vi "Versuchsaufbau bearbeiten.vi"(6 "error in (no error)":errorcluster, 8 "Setup in":refnum<class "Setup.lvclass">, 9 "Data":T1={"Report.lvclass"=refnum, "Norm"="", "last State"=enum."Initialize", "Norm ID"=0, "EMTestCWS500N.lvclass"=refnum, "CEG4500.lvclass"=refnum, "Tektronix RSA5106A.lvclass"=refnum, "erfolgreich"=FALSE, "Device Enum"=enum."emTestCWS500N", "Test Enum"=enum."ESD", "debug"=FALSE, "tab"=enum."Hauptmenü", "ESD Pistol.lvclass"=refnum, "SubPnl Refnum"=refnum, "TabCtl Refnum"=refnum, "ButtonsEinblenden?"=FALSE, "VKey"=enum."ASCII", "last Test"=refnum}) -> (0 "error out 2":errorcluster caption="error out", 2 "Setup Ausgang":refnum<class "Setup.lvclass">, 3 "Abbrechen out":bool)   [LabVIEW 2013, in "DataCreation.lvlib"]
doc: "Hier wird der Versuchsaufbau dokumentiert. Es gibt die Möglichkeit Bilder und die genutzten Geräte zu hinterlegen. Mit diesem VI kann auch ein bestehender Versuchsaufbau bearbeitet werden, in diesem Fall wird ein Setup-Objekt als Eingabe benötigt.\nNach korrekter Ausführung wird ein Setup-Objekt zurückgegeben das einem Norm-Objekt zugeordnet werden kann."
uses:
  lib/DataCreation.lvlib
  Main/controls/Data.ctl
  classes/Datastructure/Report/Report.lvclass
  classes/Devices/emTestCWS500N/EMTestCWS500N.lvclass
  classes/Devices/CEG4500/CEG4500.lvclass
  classes/Devices/Tektronix RSA5106A/Tektronix RSA5106A.lvclass
  ESD Pistol.lvclass
  classes/Datastructure/Test/Test.lvclass
  Main/controls/State.ctl
  classes/Devices/DeviceInterface/Devices.ctl
  classes/Tests/TestInterface/Tests.ctl
  Tabs.ctl
  <vilib>/event_ctls.llb/eventvkey.ctl
  classes/Datastructure/Setup/Setup.lvclass
  SetupData2.ctl
  classes/Datastructure/Device/Device.lvclass
  classes/Datastructure/Image/img.lvclass
  <vilib>/regexp/Match Regular Expression.xnode
  lib/TreeRepresentation.lvlib
panel:
  in  "dev id":i32
  in  "pic id":i32
  in  "Tab Control":enum32{"Versuchsaufbau", "Daten"}(tab)
  in  "Abbrechen":bool
  in  "Tree pics & devs":string(tree)
  out "Titel":string caption="Test"
  in  "OK Button":bool
  in  "Add picture":bool
  in  "Kommentar":string
  in  "Add Device":bool
  in  "Tree Report":string(tree)
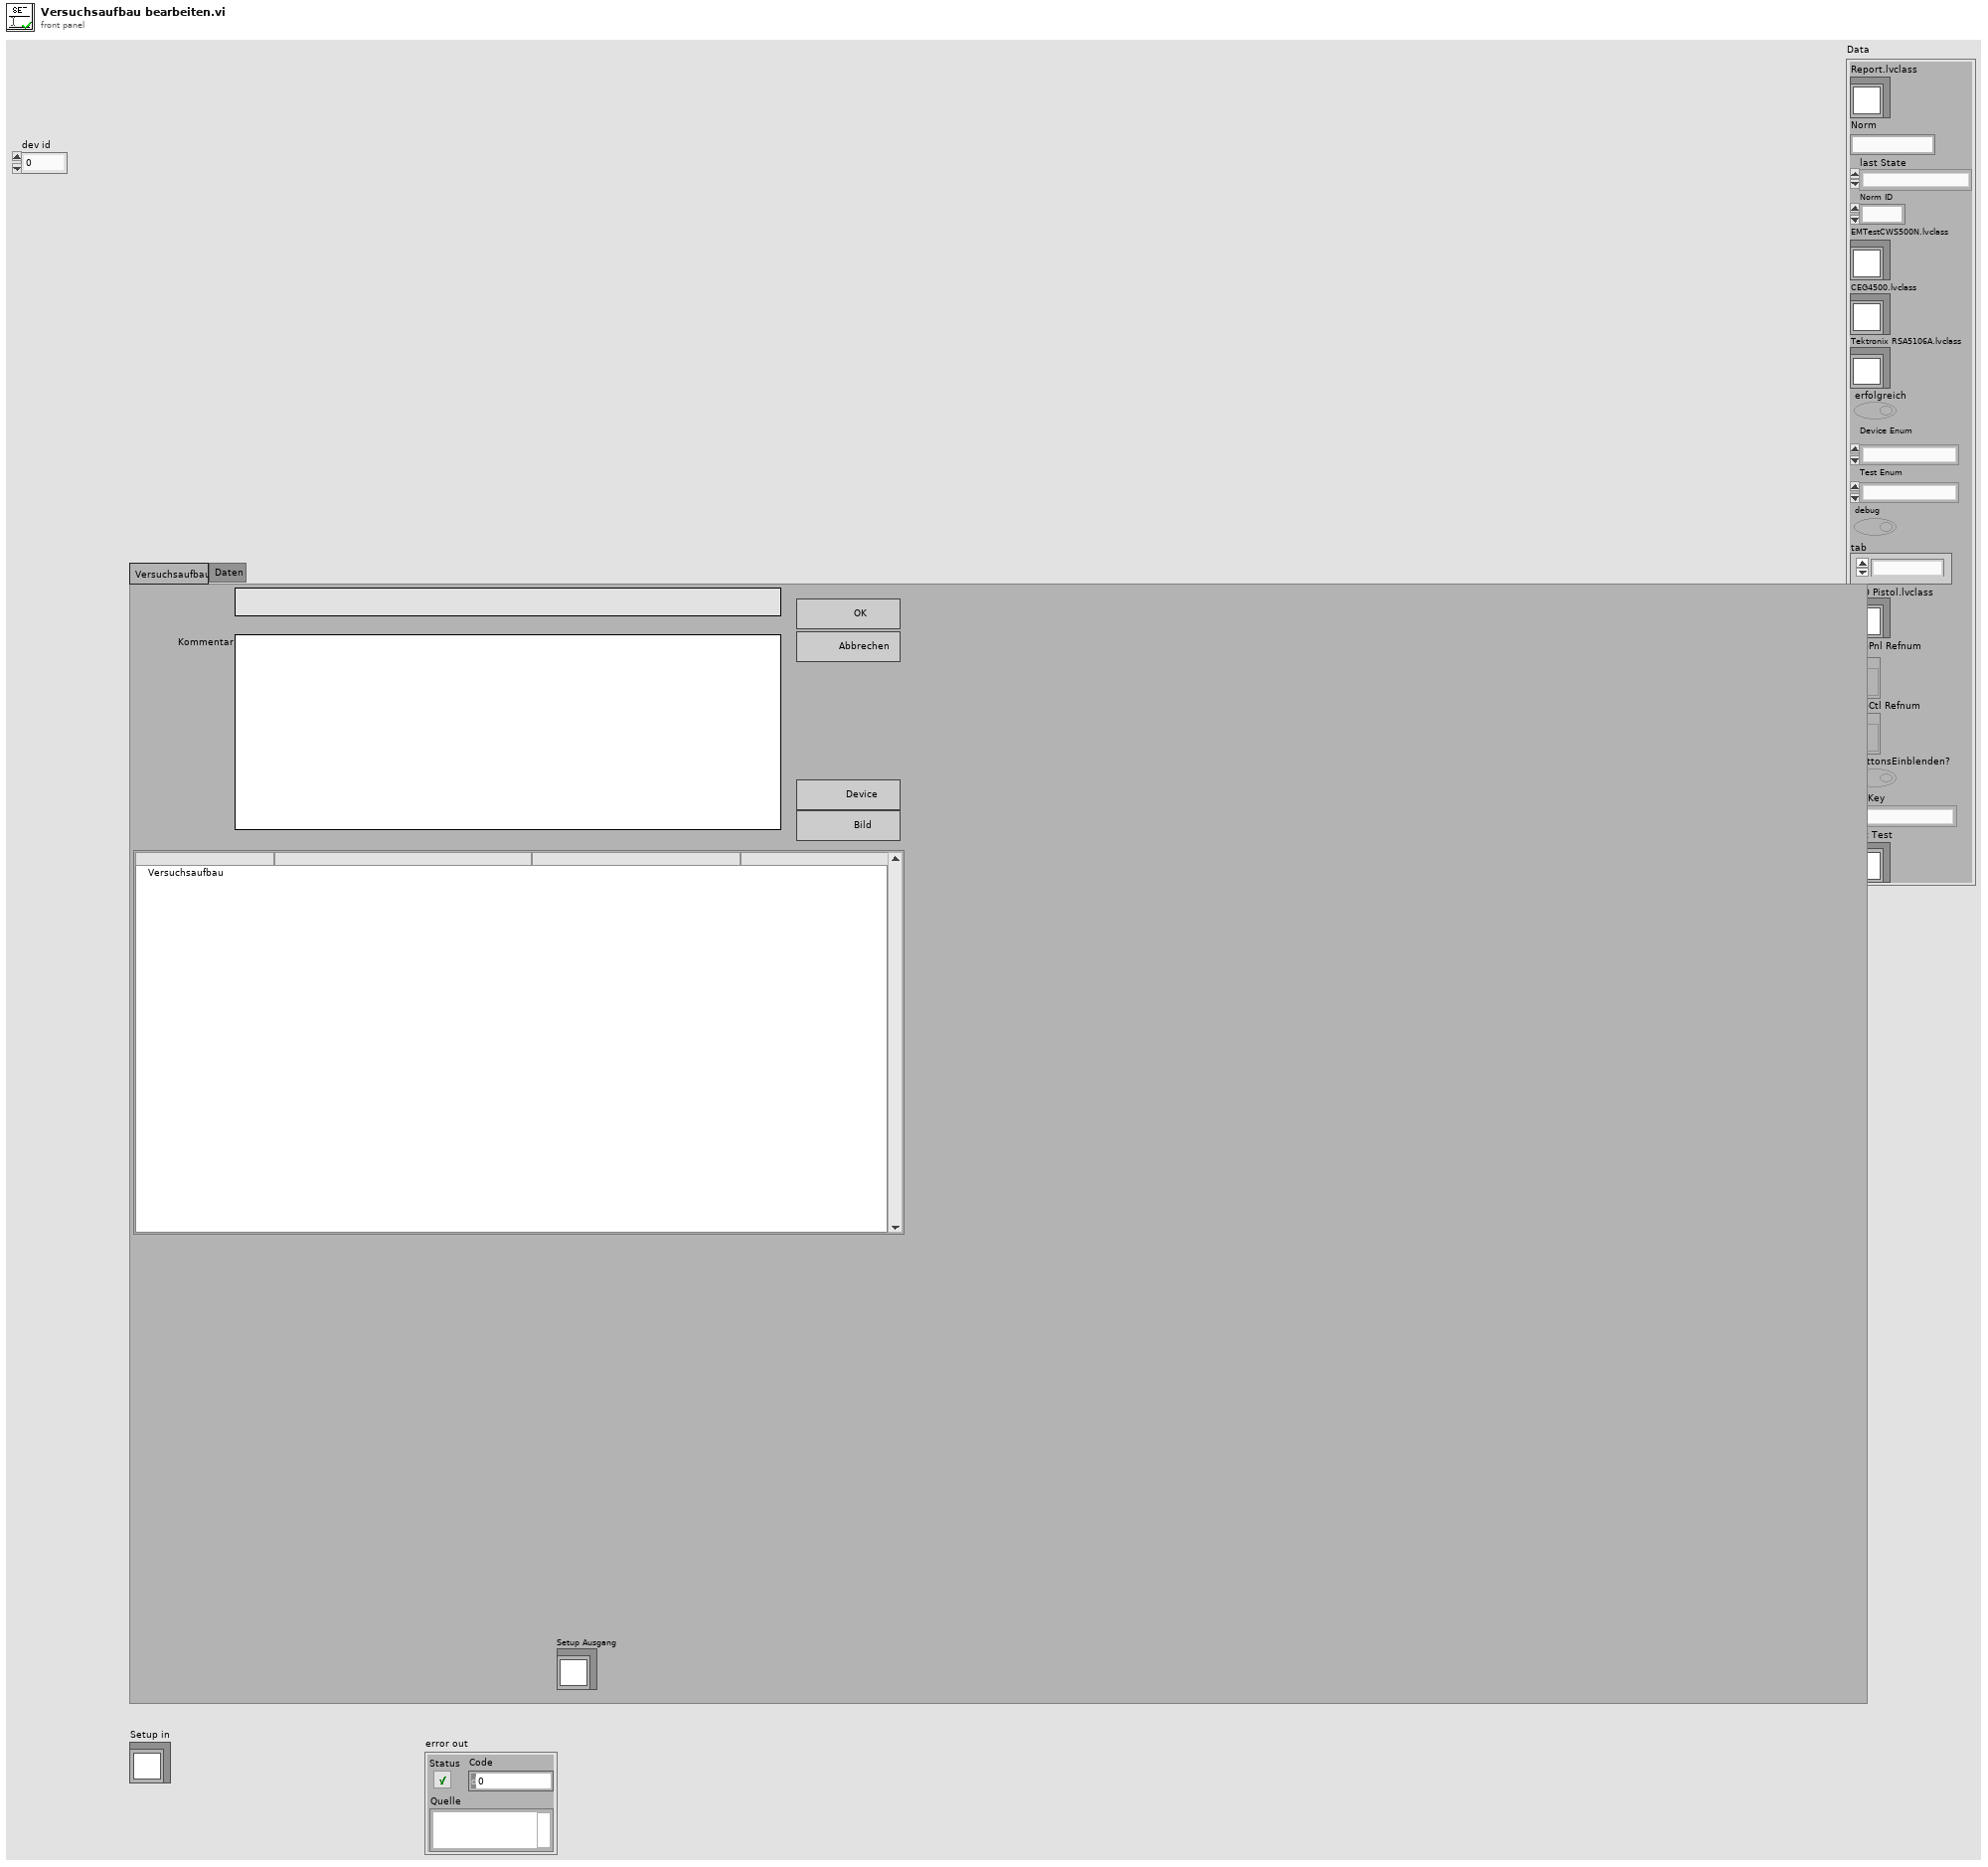
[diagram p1: front panel]
types:
  T1 = typedef "Data.ctl" = cluster{"Report.lvclass":refnum<class "Report.lvclass">, "Norm":string, "last State":T2, "Norm ID":i32, "EMTestCWS500N.lvclass":refnum<class "EMTestCWS500N.lvclass">, "CEG4500.lvclass":refnum<class "CEG4500.lvclass">, "Tektronix RSA5106A.lvclass":refnum<class "Tektronix RSA5106A.lvclass">, "erfolgreich":bool, "Device Enum":T3, "Test Enum":T4, "debug":bool, "tab":T5, "ESD Pistol.lvclass":refnum<class "ESD Pistol.lvclass">, "SubPnl Refnum":refnum<vi>, "TabCtl Refnum":refnum<vi>, "ButtonsEinblenden?":bool, "VKey":T6, "last Test":refnum<class "Test.lvclass">}
  T2 = typedef "State.ctl" = enum16{"create Pdf", "edit Report", "load Report", "save Report", "do Test", "CDN Kalibrierung", "enter Report Parameters", "new Test", "Protokoll", "read Tree", "update Tree", "Fehler", "Initialize", "Wait for Event", "Exit"}
  T3 = typedef "Devices.ctl" = enum16{"unbekannt", "ESD Pistol", "Tektronix RSA5106A", "emTestCWS500N", "CEG-4500"}
  T4 = typedef "Tests.ctl" = enum16{"unbekannt", "Störaussendung", "Burst", "ESD", "Surge", "Spannungseinbruch", "HF-Felder"}
  T5 = typedef "Tabs.ctl" = enum32{"Hauptmenü", "Prüfbericht", "Einstellungen"}
  T6 = typedef "eventvkey.ctl" = enum16{"ASCII", "Enter", "Return", "Shift", "Ctrl", "Alt", "Cmd", "Opt", "Caps", "NumLock", "Clear", "Break", "Up", "Down", "Left", "Right", "Insert", "Delete", "Home", "End", "PageUp", "PageDown", "Escape", "Help", "Pause", "ScrollLock", "F1", "F2", "F3", "F4", "F5", "F6", "F7", "F8", "F9", "F10", "F11", "F12", "F13", "F14", "F15", "F16", "F17", "F18", "F19", "F20", "F21", "F22", "F23", "F24", "Play", "VolumeUp", "VolumeDown", "Mute", "Two Byte Char"}
  T7 = typedef "DataCreation.lvlib/SetupData2.ctl" = cluster{"Device":refnum<class "Device.lvclass">, "img":refnum<class "img.lvclass">, "tag":string, "editDev":bool}
  T8 = enum16{"add pic", "add dev", "ok", "abbrechen", "wait for event"}
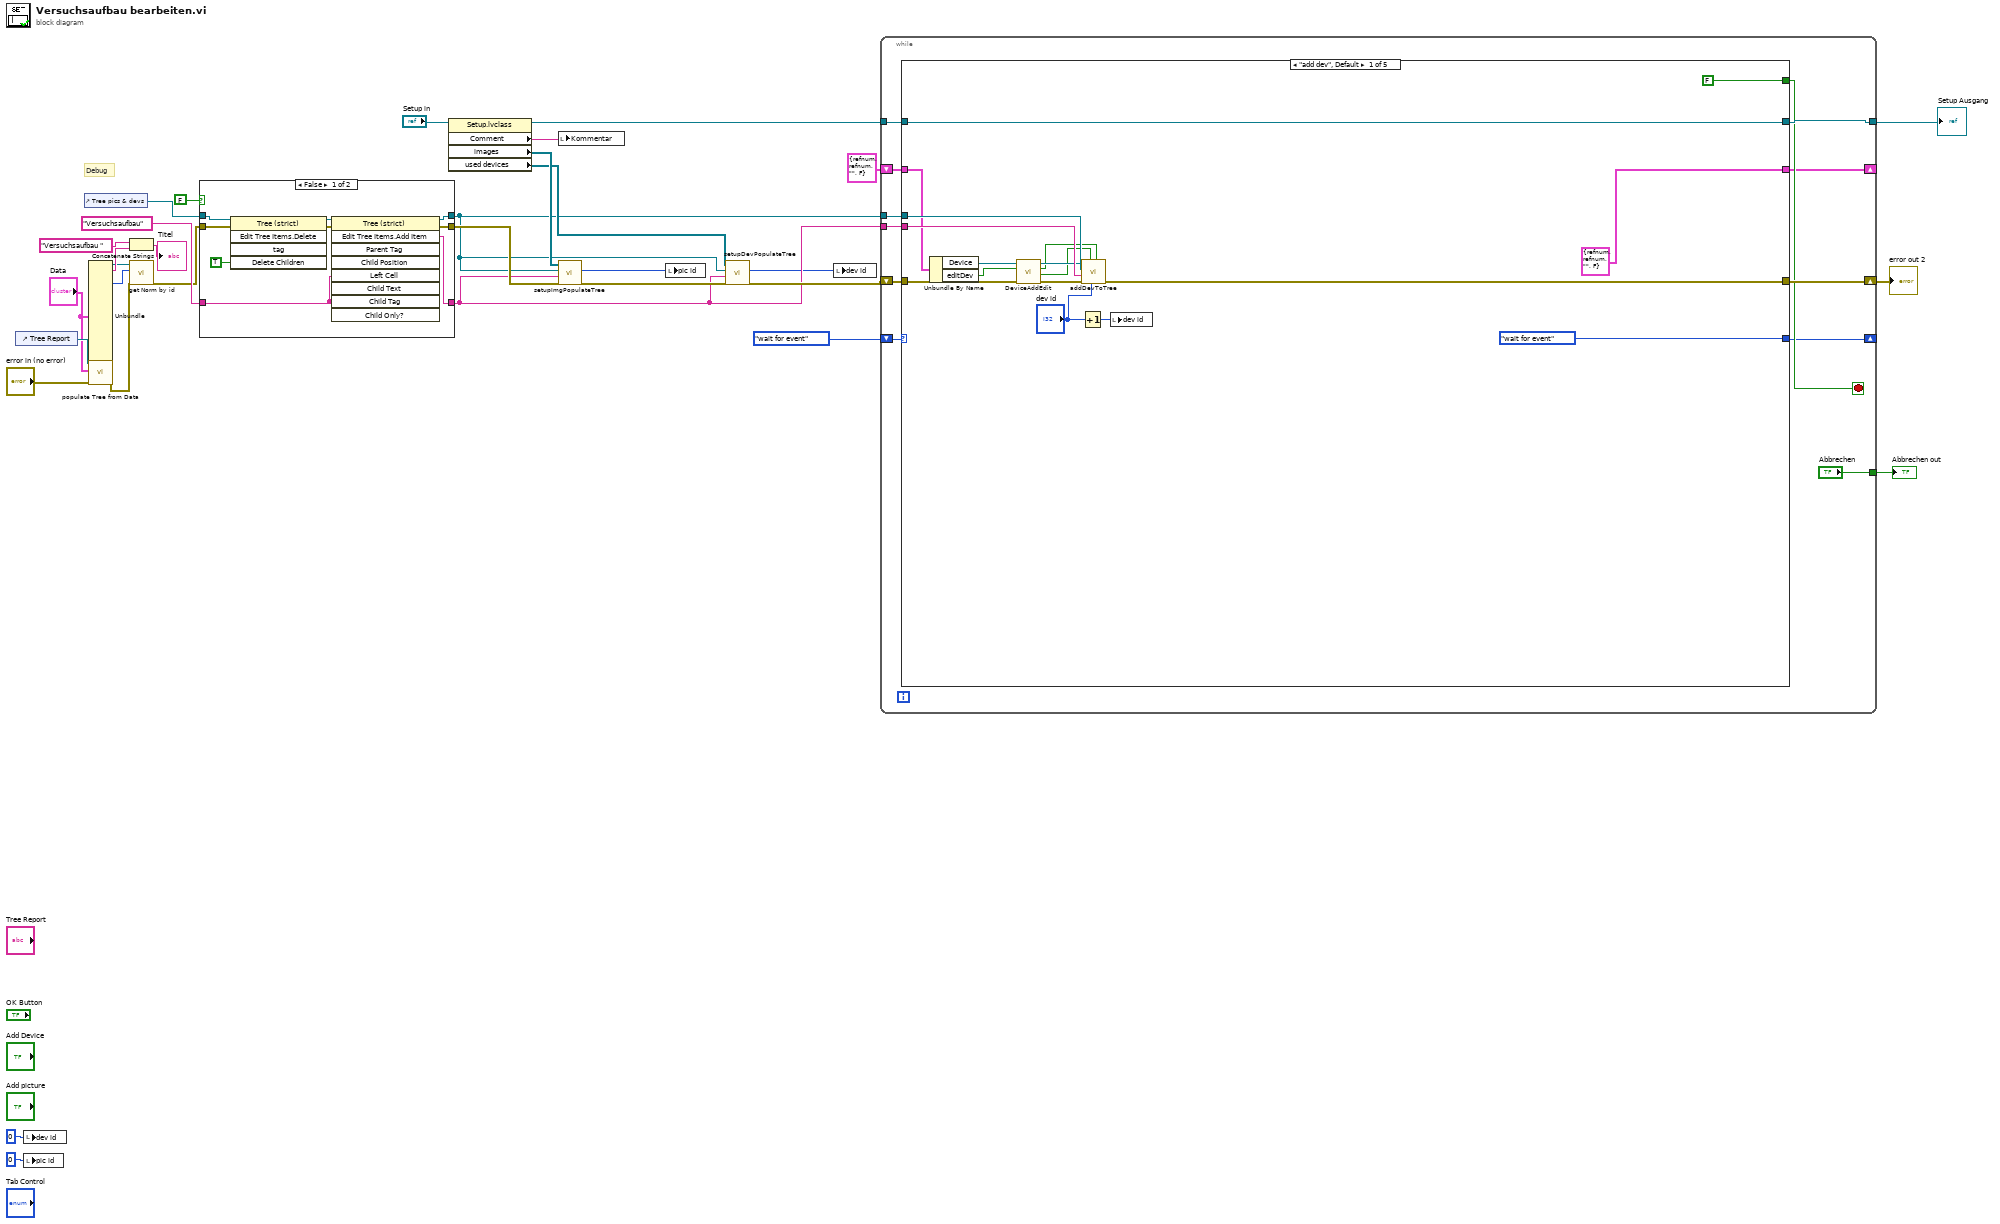
[diagram p0: block diagram]
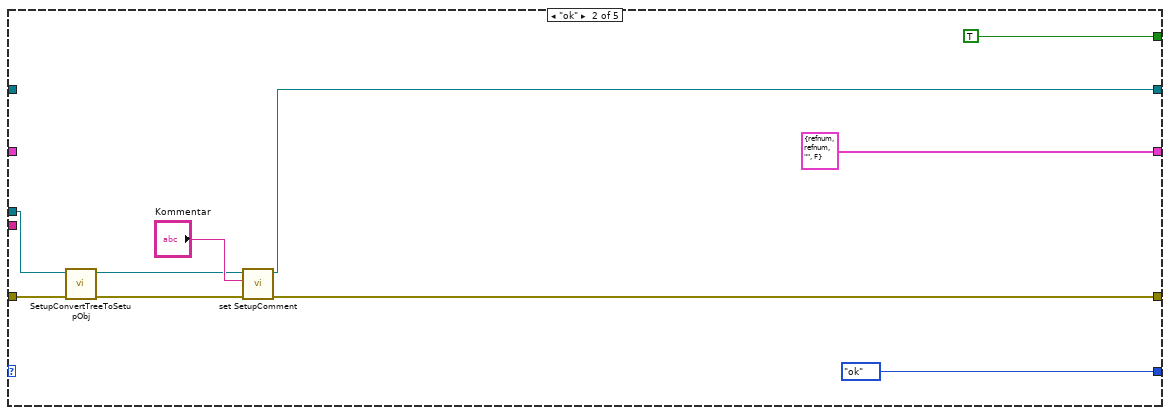
[diagram p3: hidden frame]
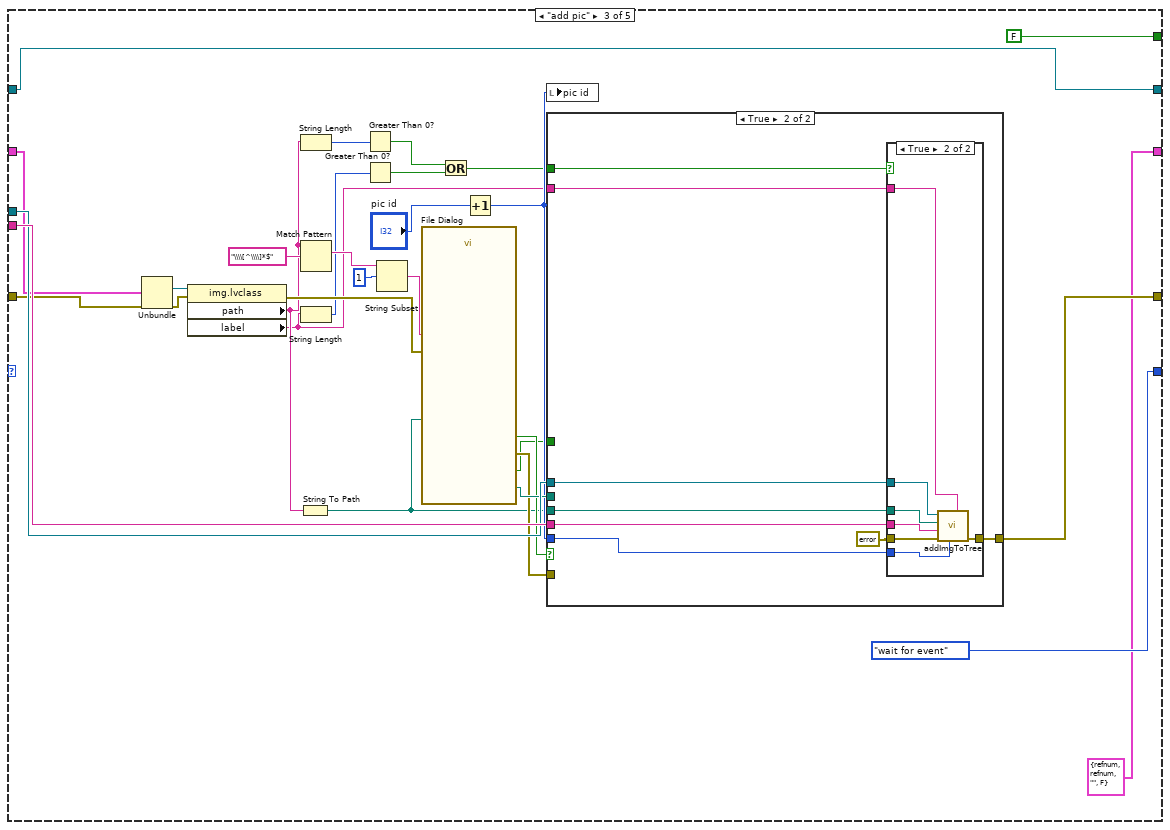
[diagram p4: hidden frame]
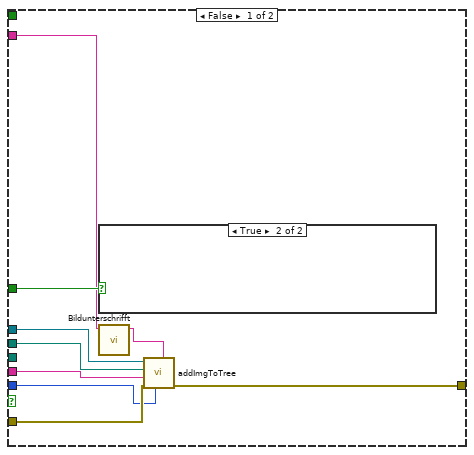
[diagram p5: hidden frame]
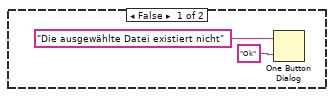
[diagram p6: hidden frame]
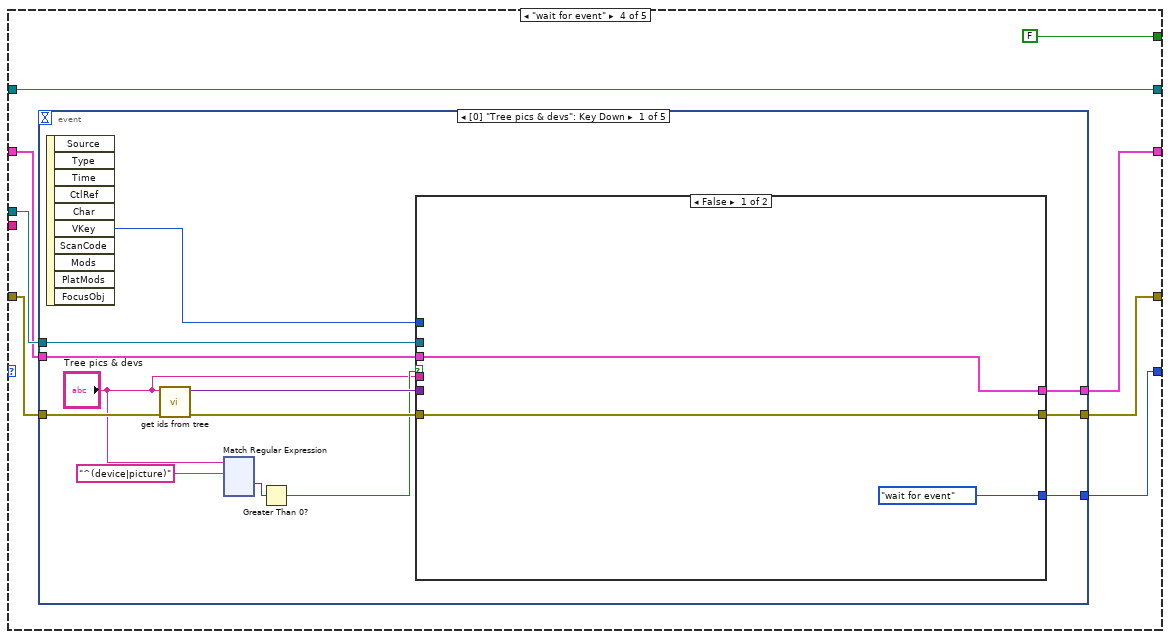
[diagram p8: hidden frame]
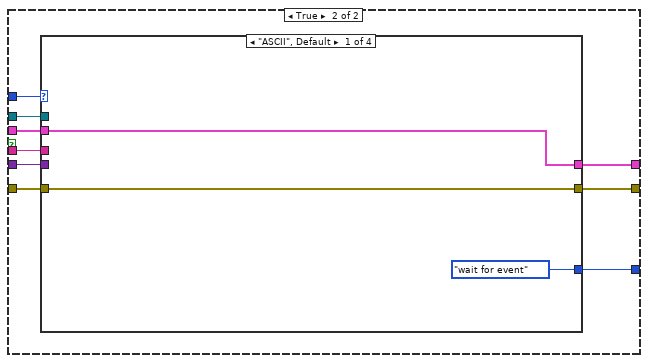
[diagram p9: hidden frame]
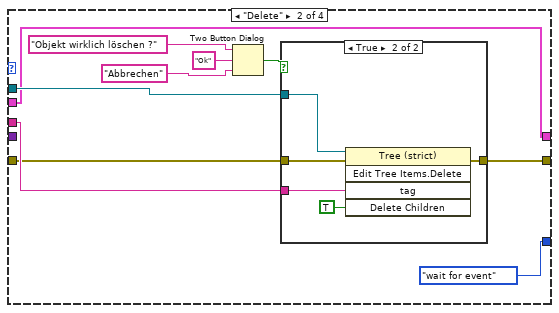
[diagram p10: hidden frame]
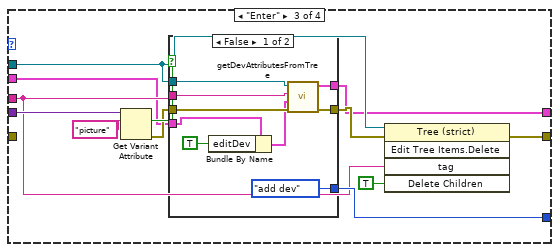
[diagram p12: hidden frame]
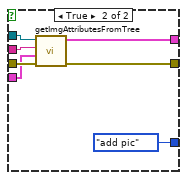
[diagram p13: hidden frame]
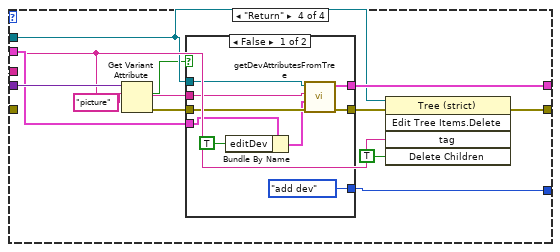
[diagram p14: hidden frame]
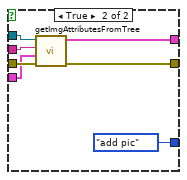
[diagram p15: hidden frame]
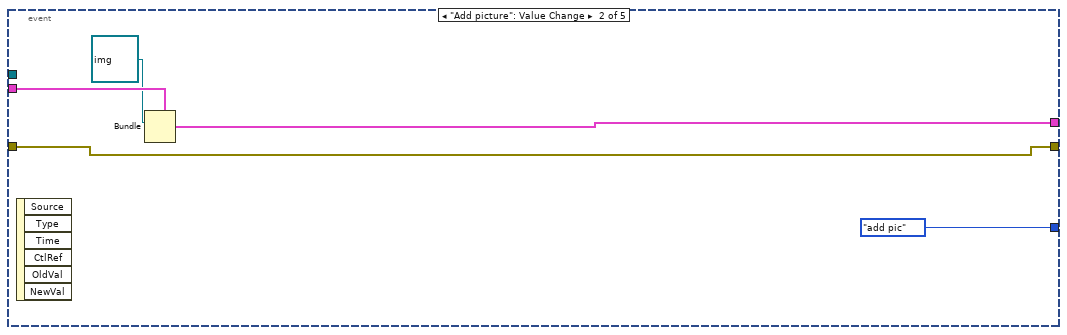
[diagram p16: hidden frame]
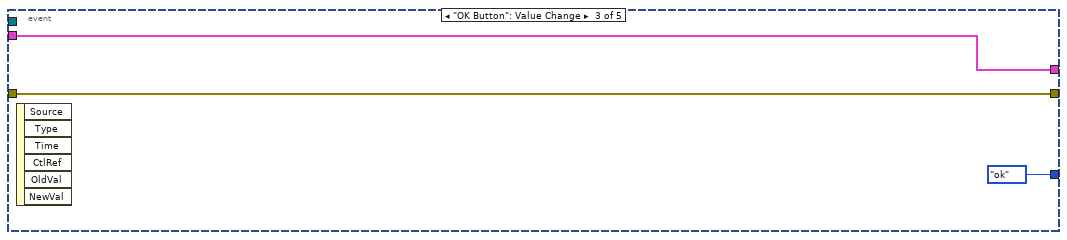
[diagram p17: hidden frame]
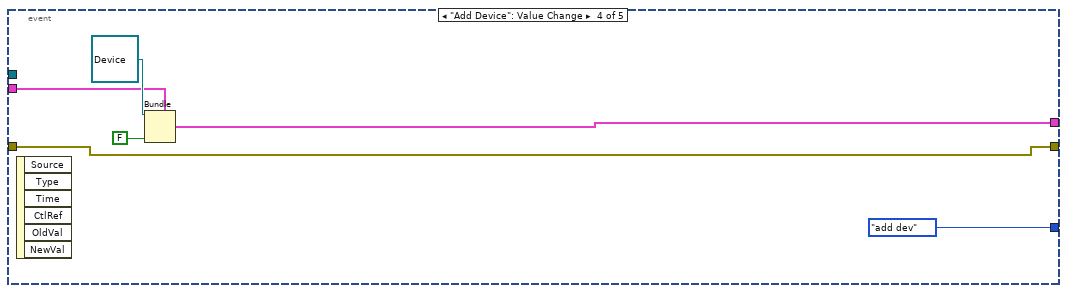
[diagram p18: hidden frame]
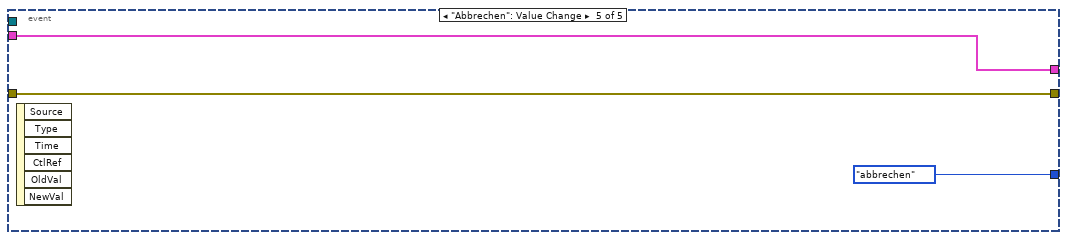
[diagram p19: hidden frame]
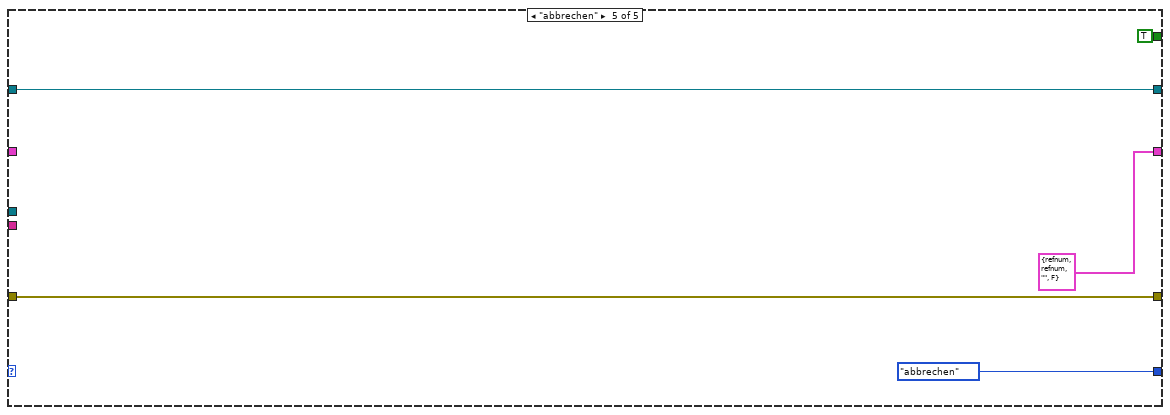
[diagram p20: hidden frame]
diagram:
  # "Debug"
  n1 = control-ref of="Tree Report"() -> (w32:refnum<vi>)
  n2 = local write "dev id"(0 ("number of devices")) -> ()
  n3 = local write "pic id"(0 ("number of devices")) -> ()
  n4 = control-ref of="Tree pics & devs"() -> (w21:refnum<vi>)
  n5 = Unbundle("Data") -> ("Report.lvclass"=w27:refnum<class "Report.lvclass">, "Norm"=w28:string, "Norm ID"=w24:i32)  [unwired: 15 out]
  n6 = call "populate Tree from Data.vi"("error in (no error)"="error in (no error)", "Data"="Data", "reference"=w32) -> ("error out"=w26:errorcluster)  [unwired: 6 in]
  n7 = Concatenate Strings("Versuchsaufbau ", w28) -> (→"Titel":string)
  n8 = call-dynamic "get Norm by id.vi"("error in (no error)"=w26, "id"=w24, "Report (Eingang)"=w27) -> ("error out"=w22:errorcluster)  [unwired: 4 in, 4 out]
  n9 = case shown="False" FALSE {
    tunnel: "Versuchsaufbau" ("Elternobjekt-Tag") -> [w41 w42]
    tunnel: [w40 w42] -> w10
    tunnel: [w39 w44] -> w15
    tunnel: w22 -> [w38 w44]
    tunnel: w21 -> [w37 w43]
    tunnel: [w36 w43] -> w8
    frame False {
      n10 = invoke on="Invoke Node" class="Tree (strict)" method="Edit Tree Items.Delete"(reference=w37, error in=w38, "Delete Children"=TRUE ("Unterobjekte löschen?")) -> (reference out=w35:refnum<vi>, error out=w34:errorcluster)  [unwired: 2 in, 3 out]
      n11 = invoke class="Tree (strict)" method="Edit Tree Items.Add Item"(reference=w35, error in=w34, "Left Cell"=w41, "Child Tag"=w41) -> (reference out=w36:refnum<vi>, error out=w39:errorcluster, "Edit Tree Items:Add Item"=w40:string)  [unwired: 5 in, 6 out]
    }
    frame True {
    }
  }
  n12 = property class="Setup.lvclass"(reference="Setup in") -> (reference out=w5:refnum<class "Setup.lvclass">, "Comment"=w16:string, "images"=w13:refnum<class "img.lvclass">[], "used devices"=w9:refnum<class "Device.lvclass">[])  [unwired: 1 in, 1 out]
  n13 = local write "Kommentar"(w16) -> ()
  n14 = call "setupImgPopulateTree.vi"("error in (no error)"=w15, "Elternobjekt-Tag"=w10, "Tree in"=w8, "images"=w13) -> ("error out"=w12:errorcluster, "#pics"=w14:i32)  [unwired: 6 in]
  n15 = local write "pic id"(w14) -> ()
  n16 = call "setupDevPopulateTree.vi"("error in (no error)"=w12, "Elternobjekt-Tag"=w10, "TreeControl in"=w8, "used devices"=w9) -> ("error out"=w11:errorcluster, "#dev"=w7:i32)  [unwired: 6 in]
  n17 = local write "dev id"(w7) -> ()
  n18 = while {
    tunnel: w10 -> [w53]
    tunnel: w8 -> [w55]
    tunnel: [w52] -> w3
    shift-right: [w51] -> w4
    shift-left: w11 -> [w56]
    shift-right: [w49] -> _
    shift-left: T8."wait for event" -> [w54]
    tunnel: w5 -> [w48]
    shift-right: [w46] -> _
    shift-left: T7 {"Device"=refnum, "img"=refnum, "tag"="", "editDev"=FALSE} -> [w47]
    tunnel: ["Abbrechen"] -> w1
    stop <- w50 stop-if-true
    n19 = case shown="\"add dev\", Default" w54 {
      tunnel: [w71 w75 w112 w141 w381] -> w51
      tunnel: w56 -> [w64 w82 w102 w142 w381]
      tunnel: w53 -> [w73 _ w111 _ _]
      tunnel: w55 -> [w72 w83 w110 w147 _]
      tunnel: [w68 w76 w105 w144 w380] -> w52
      tunnel: [FALSE TRUE FALSE FALSE TRUE] -> w50
      tunnel: [T8."wait for event" T8."ok" T8."wait for event" w145 T8."abbrechen"] -> w49
      tunnel: w48 -> [w68 _ w105 w144 w380]
      tunnel: w47 -> [w67 _ w104 w143 _]
      tunnel: [T7 {"Device"=refnum, "img"=refnum, "tag"="", "editDev"=FALSE} T7 {"Device"=refnum, "img"=refnum, "tag"="", "editDev"=FALSE} T7 {"Device"=refnum, "img"=refnum, "tag"="", "editDev"=FALSE} w140 T7 {"Device"=refnum, "img"=refnum, "tag"="", "editDev"=FALSE}] -> w46
      frame "add dev", Default {
        n20 = Unbundle By Name(w67) -> ("Device"=w66:refnum<class "Device.lvclass">, "editDev"=w57:bool)
        n21 = call "DeviceAddEdit.vi"("error in"=w64, "editDev"=w57, "Dev in"=w66) -> ("error out"=w63:errorcluster, "Dev löschen"=w62:bool, "Abbruch?"=w58:bool, "Dev out"=w65:refnum<class "Device.lvclass">)  [unwired: 5 in]
        n22 = Increment(x="dev id") -> (x+1=w59:i32)
        n23 = call "addDevToTree.vi"("abbrechen"=w58, "dev id"="dev id", "Dev löschen"=w62, "error in (no error)"=w63, "Elternobjekt-Tag"=w73, "Tree pics & devs"=w72, "Device in"=w65) -> ("error out"=w71:errorcluster)  [unwired: 4 in]
        n24 = local write "dev id"(w59) -> ()
      }
      frame "ok" {
        n25 = call "SetupConvertTreeToSetupObj.vi"("error in (no error)"=w82, "TreeControl in"=w83) -> ("error out"=w79:errorcluster, "Setup out"=w77:refnum<class "Setup.lvclass">)  [unwired: 8 in]
        n26 = call-dynamic "set SetupComment.vi"("error in (no error)"=w79, "Comment"="Kommentar", "Setup (Eingang)"=w77) -> ("error out"=w75:errorcluster, "Setup (Ausgang)"=w76:refnum<class "Setup.lvclass">)  [unwired: 7 in]
      }
      frame "add pic" {
        n27 = Unbundle(w104) -> ("img"=w103:refnum<class "img.lvclass">)  [unwired: 3 out]
        n28 = property class="img.lvclass"(reference=w103, error in=w102) -> (error out=w101:errorcluster, "path"=w93:string, "label"=w92:string)  [unwired: 1 out]
        n29 = String To Path(string=w93) -> (path=w86:path)
        n30 = String Length(string=w93) -> (length=w91:i32)
        n31 = Match Pattern(string=w93, regular expression="\\\\[^\\\\]*$") -> (match substring=w96:string)  [unwired: 1 in, 3 out]
        n32 = String Length(string=w92) -> (length=w90:i32)
        n33 = Greater Than 0?(x=w91) -> (x > 0?=w89:bool)
        n34 = Greater Than 0?(x=w90) -> (x > 0?=w88:bool)
        n35 = String Subset(string=w96, offset (0)=1) -> (substring=w94:string)  [unwired: 1 in]
        n36 = call "File Dialog"("start path"=w86, "default name"=w94, "error in"=w101) -> ("selected path"=w109:path, "exists"=w84:bool, "cancelled"=w87:bool, "error out"=w108:errorcluster)  [unwired: 9 in]
        n37 = Or(x=w89, y=w88) -> (x .or. y?=w85:bool)
        n38 = Increment(x="pic id") -> (x+1=w98:i32)
        n39 = local write "pic id"(w98) -> ()
        n40 = case shown="True" w87 {
          tunnel: [w121 w125] -> w112
          tunnel: w111 -> [w120 w130]
          tunnel: w110 -> [w119 w128]
          tunnel: w109 -> [w118 _]
          tunnel: w108 -> [w117 _]
          tunnel: w98 -> [w116 w129]
          tunnel: w92 -> [w114 w126]
          tunnel: w86 -> [_ w131]
          tunnel: w85 -> [_ w127]
          tunnel: w84 -> [w115 _]
          frame False {
            n41 = case shown="True" w115 {
              frame False {
                n42 = One Button Dialog(message="Die ausgewählte Datei existiert nicht", button name ("OK")="Ok") -> ()  [unwired: 1 out]
              }
              frame True {
              }
            }
            n43 = call "Bildunterschrifft.vi"("Bildunterschrifft"=w114) -> ("Bildunterschrifft out"=w113:string)  [unwired: 10 in]
            n44 = call "addImgToTree.vi"("Bildunterschrifft"=w113, "Numeric"=w116, "error in (no error)"=w117, "Elternobjekt-Tag"=w120, "selected path"=w118, "TreeControl in"=w119) -> ("error out"=w121:errorcluster)  [unwired: 5 in]
          }
          frame True {
            n45 = case shown="True" w127 {
              tunnel: w131 -> [_ w136]
              tunnel: errorcluster {"status"=FALSE, "code"=0, "source"=""} ("error out") -> [w132 w139]
              tunnel: w130 -> [_ w138]
              tunnel: w129 -> [_ w137]
              tunnel: w128 -> [_ w135]
              tunnel: w126 -> [_ w134]
              tunnel: [w132 w133] -> w125
              frame False {
              }
              frame True {
                n46 = call "addImgToTree.vi"("Bildunterschrifft"=w134, "Numeric"=w137, "error in (no error)"=w139, "Elternobjekt-Tag"=w138, "selected path"=w136, "TreeControl in"=w135) -> ("error out"=w133:errorcluster)  [unwired: 5 in]
              }
            }
          }
        }
      }
      frame "wait for event" {
        n47 = event shown="[0] \"Tree pics & devs\": Key Down" {
          selector: _ -> [_ _ _ _ _]
          dyn-events: _ -> [_ _ _ _ _]
          timeout: _ -> [_ _ _ _ _]
          tunnel: w147 -> [w159 _ _ _ _]
          tunnel: [w158 T8."add pic" T8."ok" T8."add dev" T8."abbrechen"] -> w145
          tunnel: w143 -> [w153 w363 w367 w371 w376]
          tunnel: w142 -> [w157 w365 w368 w372 w377]
          tunnel: [w154 w365 w368 w372 w377] -> w141
          tunnel: [w152 w364 w367 w373 w376] -> w140
          event "Tree pics & devs": Key Down {
            n48 = event-data() -> ("VKey"=w160:T6)  [unwired: 1 in, 9 out]
            n49 = call "get ids from tree.vi"("error in"=w157, "Tree"="Tree pics & devs") -> ("error out"=w155:errorcluster, "tags"=w156:variant)  [unwired: 8 in]
            n50 = xnode "Match Regular Expression"("input string"="Tree pics & devs", "regular expression"="^(device|picture)") -> ("offset past match"=w148:i32)  [unwired: 4 in, 4 out]
            n51 = Greater Than 0?(x=w148) -> (x > 0?=w151:bool)
            n52 = case shown="False" w151 {
              tunnel: w160 -> [_ w286]
              tunnel: w159 -> [_ w285]
              tunnel: [T8."wait for event" w284] -> w158
              tunnel: "Tree pics & devs" -> [_ w283]
              tunnel: w156 -> [_ w282]
              tunnel: w155 -> [w277 w281]
              tunnel: [w277 w280] -> w154
              tunnel: w153 -> [w276 w279]
              tunnel: [w276 w278] -> w152
              frame False {
              }
              frame True {
                n53 = case shown="\"ASCII\", Default" w286 {
                  tunnel: w285 -> [_ w299 w310 w335]
                  tunnel: w283 -> [_ w298 w311 w336]
                  tunnel: [T8."wait for event" T8."wait for event" w317 w341] -> w284
                  tunnel: w282 -> [_ _ w316 w345]
                  tunnel: w281 -> [w289 w292 _ _]
                  tunnel: [w289 w291 w312 w342] -> w280
                  tunnel: w279 -> [w287 w290 w307 w337]
                  tunnel: [w287 w290 w306 w339] -> w278
                  frame "ASCII", Default {
                  }
                  frame "Delete" {
                    n54 = Two Button Dialog(message="Objekt wirklich löschen ?", 1:"Abbrechen" ("F button name (\"Cancel\")"), 2:"Ok" ("T button name (\"OK\")")) -> (T button?=w294:bool)
                    n55 = case shown="True" w294 {
                      tunnel: w299 -> [_ w305]
                      tunnel: w298 -> [_ w303]
                      tunnel: w292 -> [w300 w302]
                      tunnel: [w300 w301] -> w291
                      frame False {
                      }
                      frame True {
                        n56 = invoke class="Tree (strict)" method="Edit Tree Items.Delete"(reference=w305, error in=w302, "tag"=w303, "Delete Children"=TRUE ("Delete Children?")) -> (error out=w301:errorcluster)  [unwired: 1 in, 4 out]
                      }
                    }
                  }
                  frame "Enter" {
                    n57 = Get Variant Attribute(Variant=w316, name="picture") -> (found=w314:bool, error out=w309:errorcluster)  [unwired: 2 in, 2 out]
                    n58 = case shown="False" w314 {
                      tunnel: [T8."add dev" T8."add pic"] -> w317
                      tunnel: w311 -> [w325 w328]
                      tunnel: w310 -> [w324 w329]
                      tunnel: w309 -> [w323 w332]
                      tunnel: [w322 w331] -> w308
                      tunnel: w307 -> [w320 w327]
                      tunnel: [w321 w330] -> w306
                      frame False {
                        n59 = Bundle By Name(cluster=w320, "editDev"=TRUE) -> (w318:T7)
                        n60 = call "getDevAttributesFromTree.vi"("error in (no error)"=w323, "Cluster in"=w318, "Tree pics & devs in"=w325, "TreeControl in"=w324) -> ("error out"=w322:errorcluster, "Cluster out"=w321:T7)  [unwired: 6 in]
                      }
                      frame True {
                        n61 = call "getImgAttributesFromTree.vi"("error in (no error)"=w332, "Cluster in"=w327, "Tree pics & devs in"=w328, "TreeControl in"=w329) -> ("error out"=w331:errorcluster, "Cluster out"=w330:T7)  [unwired: 6 in]
                      }
                    }
                    n62 = invoke class="Tree (strict)" method="Edit Tree Items.Delete"(reference=w310, error in=w308, "tag"=w311, "Delete Children"=TRUE ("Delete Children?")) -> (error out=w312:errorcluster)  [unwired: 1 in, 4 out]
                  }
                  frame "Return" {
                    n63 = Get Variant Attribute(Variant=w345, name="picture") -> (found=w334:bool, error out=w338:errorcluster)  [unwired: 2 in, 2 out]
                    n64 = case shown="False" w334 {
                      tunnel: [T8."add dev" T8."add pic"] -> w341
                      tunnel: w336 -> [w353 w356]
                      tunnel: w335 -> [w352 w357]
                      tunnel: w338 -> [w351 w360]
                      tunnel: [w350 w359] -> w340
                      tunnel: w337 -> [w348 w355]
                      tunnel: [w349 w358] -> w339
                      frame False {
                        n65 = Bundle By Name(cluster=w348, "editDev"=TRUE) -> (w346:T7)
                        n66 = call "getDevAttributesFromTree.vi"("error in (no error)"=w351, "Cluster in"=w346, "Tree pics & devs in"=w353, "TreeControl in"=w352) -> ("error out"=w350:errorcluster, "Cluster out"=w349:T7)  [unwired: 6 in]
                      }
                      frame True {
                        n67 = call "getImgAttributesFromTree.vi"("error in (no error)"=w360, "Cluster in"=w355, "Tree pics & devs in"=w356, "TreeControl in"=w357) -> ("error out"=w359:errorcluster, "Cluster out"=w358:T7)  [unwired: 6 in]
                      }
                    }
                    n68 = invoke class="Tree (strict)" method="Edit Tree Items.Delete"(reference=w335, error in=w340, "tag"=w336, "Delete Children"=TRUE ("Delete Children?")) -> (error out=w342:errorcluster)  [unwired: 1 in, 4 out]
                  }
                }
              }
            }
          }
          event "Add picture": Value Change {
            n69 = event-data() -> ()  [unwired: 1 in, 6 out]
            n70 = Bundle(cluster=w363, "img"=refnum<class "img.lvclass"> refnum) -> (w364:T7)  [unwired: 3 in]
          }
          event "OK Button": Value Change {
            n71 = event-data() -> ()  [unwired: 1 in, 6 out]
          }
          event "Add Device": Value Change {
            n72 = event-data() -> ()  [unwired: 1 in, 6 out]
            n73 = Bundle(cluster=w371, "Device"=refnum<class "Device.lvclass"> refnum, "editDev"=FALSE) -> (w373:T7)  [unwired: 2 in]
          }
          event "Abbrechen": Value Change {
            n74 = event-data() -> ()  [unwired: 1 in, 6 out]
          }
        }
      }
      frame "abbrechen" {
      }
    }
  }
  "error out 2" <- w4
  "Setup Ausgang" <- w3
  "Abbrechen out" <- w1
